vi "Teleop.vi"(9 "Inputs":T7, 10 "Match Info":T12={"Autonomous Elapsed Seconds"=0.0, "TeleOp Elapsed Seconds"=0.0, "Disabled Elapsed Seconds"=0.0, "Visited Autonomous"=FALSE, "Visited TeleOp"=FALSE, "Visited Disabled"=FALSE, "Autonomous Settings"={"Autonomous Style"=enum."Independent", "VI Refnum"=refnum}}, 11 "Call Context":T13) -> (3 "Outputs":T1)   [LabVIEW 2013]
doc: "This VI is called for each TeleOp packet received from the DS where the robot is not disabled. It is often used to read from the joysticks and update I/O or to update setpoints for timed control loops. It should complete and return within 20 milliseconds or it may miss DS packets."
uses:
  <vilib>/Rock Robotics/WPI/DriverStation/WPI_DriverStationDerivedRobotMode.ctl
  <vilib>/Rock Robotics/WPI/DriverStation/WPI_DriverStationMatch Info.ctl
  util/inputs.ctl
  drive/drive_inputs.ctl
  flinger/flinger_inputs.ctl
  roller/roller_inputs.ctl
  catch/catch_inputs.ctl
  util/outputs.ctl
  drive/drive_outputs.ctl
  flinger/flinger_outputs.ctl
  <vilib>/Rock Robotics/WPI/Solenoid/WPI_SolenoidValue.ctl
  roller/roller_outputs.ctl
  catch/catch_outputs.ctl
  Robot Global Data.vi
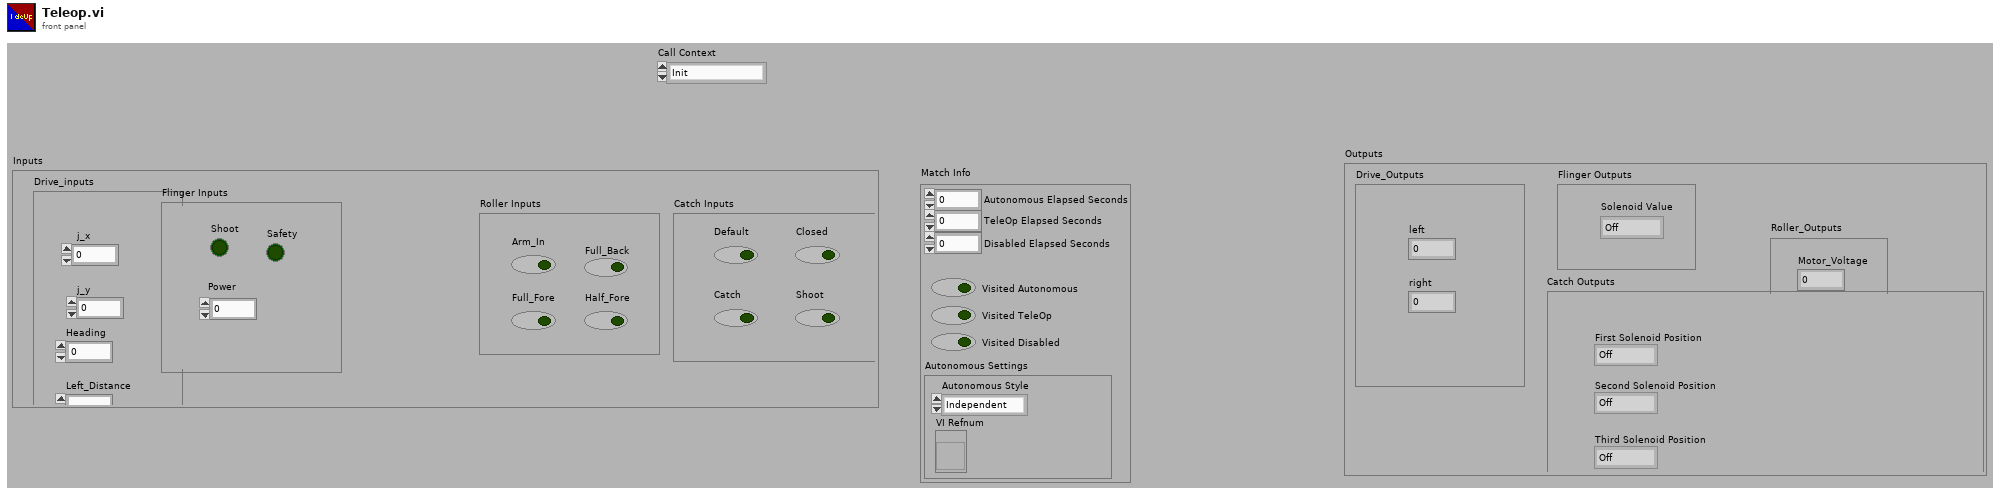
[diagram p1: front panel]
types:
  T1 = typedef "outputs.ctl" = cluster{"Drive_Outputs":T2, "Flinger Outputs":T3, "Roller_Outputs":T5, "Catch Outputs":T6}
  T2 = typedef "drive_outputs.ctl" = cluster{"left":dbl, "right":dbl}
  T3 = typedef "flinger_outputs.ctl" = cluster{"Solenoid Value":T4}
  T4 = typedef "WPI_SolenoidValue.ctl" = enum16{"Off", "On", "Forward", "Reverse"}
  T5 = typedef "roller_outputs.ctl" = cluster{"Sol_Position":T4, "Motor_Voltage":dbl}
  T6 = typedef "catch_outputs.ctl" = cluster{"First Solenoid Position":T4, "Second Solenoid Position":T4, "Third Solenoid Position":T4}
  T7 = typedef "inputs.ctl" = cluster{"Drive_inputs":T8, "Flinger Inputs":T9, "Roller Inputs":T10, "Catch Inputs":T11}
  T8 = typedef "drive_inputs.ctl" = cluster{"j_x":dbl, "j_y":dbl, "Heading":dbl, "Left_Distance":dbl, " Right_Distance":dbl}
  T9 = typedef "flinger_inputs.ctl" = cluster{"Shoot":bool, "Power":dbl, "Safety":bool}
  T10 = typedef "roller_inputs.ctl" = cluster{"Arm_In":bool, "Full_Fore":bool, "Full_Back":bool, "Half_Fore":bool}
  T11 = typedef "catch_inputs.ctl" = cluster{"Default":bool, "Closed":bool, "Catch":bool, "Shoot":bool}
  T12 = typedef "WPI_DriverStationMatch Info.ctl" = cluster{"Autonomous Elapsed Seconds":dbl, "TeleOp Elapsed Seconds":dbl, "Disabled Elapsed Seconds":dbl, "Visited Autonomous":bool, "Visited TeleOp":bool, "Visited Disabled":bool, "Autonomous Settings":cluster{"Autonomous Style":enum16{"Iterative", "Independent"}, "VI Refnum":refnum<vi>}}
  T13 = typedef "WPI_DriverStationDerivedRobotMode.ctl" = enum16{"Init", "Execute", "Stop"}
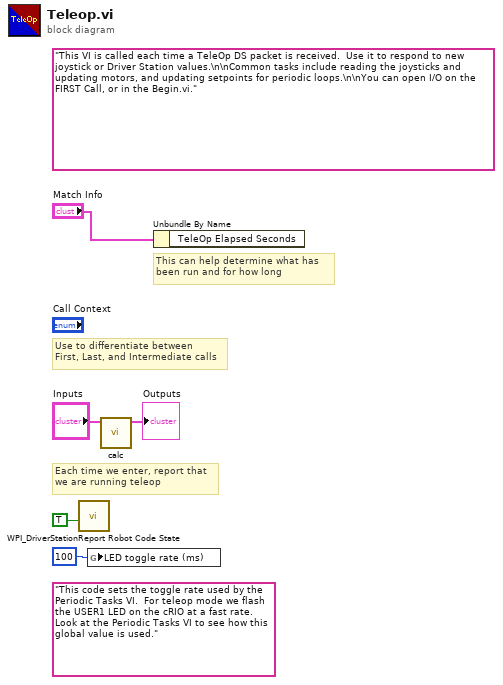
[diagram p0: block diagram]
diagram:
  (unwired) "This code sets the toggle rate used by the Periodic Tasks VI.  For teleop mode we flash the USER1 LED on the cRIO at a fast rate.  Look at the Periodic Tasks VI to see how this global value is used."
  (unwired) "This VI is called each time a TeleOp DS packet is received.  Use it to respond to new joystick or Driver Station values.\n\nCommon tasks include reading the joysticks and updating motors, and updating setpoints for periodic loops.\n\nYou can open I/O on the FIRST Call, or in the Begin.vi."
  # "Each time we enter, report that\nwe are running teleop"
  # "Use to differentiate between\nFirst, Last, and Intermediate calls"
  # "This can help determine what has\nbeen run and for how long"
  n1 = call <vilib>:"WPI_DriverStationReport Robot Code State.vi"("TeleOp"=TRUE ("Autonomous")) -> ()  [unwired: 10 in, 1 out]
  n2 = global write "Robot Global Data.vi" "LED toggle rate (ms)"(u32 100 ("LED ms toggle rate")) -> ()
  n3 = call "calc.vi"("Inputs"="Inputs") -> ("Outputs"=→"Outputs":T1)  [unwired: 10 in]
  n4 = Unbundle By Name("Match Info") -> ()  [unwired: 1 out]
